vi "Origin.vi"(0 "PortNumber":u8=7) -> (1 "Received String1":string="NG\r\n", 2 "Received String2":string, 3 "OK Done":bool)   [LabVIEW 2013]
panel:
  out "Received String Z 1":string="OK\r\n"
  in  "PortNumber Z":u8=8
  out "Received String Z 2":string
  out "OK Done Z":bool
  # "Port Number 0=COM1"
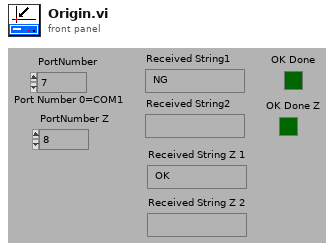
[diagram p1: front panel]
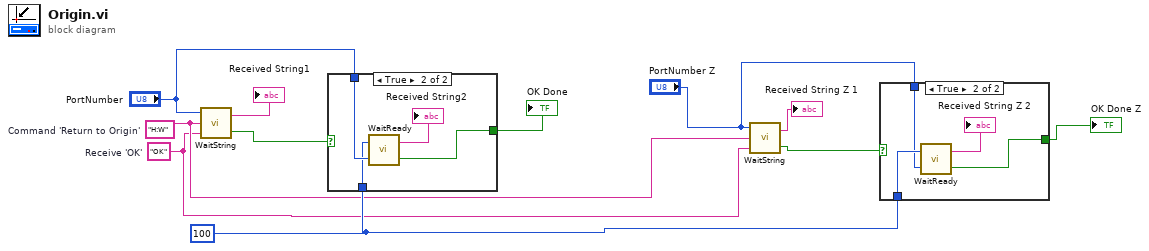
[diagram p0: block diagram]
diagram:
  w11 = 100
  w9 = "OK"  # Receive 'OK'
  w10 = "H:W"  # Command 'Return to Origin'
  n1 = call "WaitString.vi"("String to Receive"=w9, "String to Send"=w10, "PortNumber"="PortNumber") -> ("OK Done"=w5:bool, "String Received"=→"Received String1":string)
  n2 = case shown="True" w5 {
    selector: w5 -> [w12 _]
    tunnel: "PortNumber" -> [_ w16]
    tunnel: [w12 w14] -> w8
    tunnel: w11 -> [_ w13]
    frame False {
    }
    frame True {
      n3 = call "WaitReady.vi"("PortNumber"=w16, "Residence time in ms"=w13) -> ("OK Done"=w14:bool, "String Received"=→"Received String2":string)
    }
  }
  "OK Done" <- w8
  n4 = call "WaitString.vi"("String to Receive"=w9, "String to Send"=w10, "PortNumber"="PortNumber Z") -> ("OK Done"=w3:bool, "String Received"=→"Received String Z 1":string)
  n5 = case shown="True" w3 {
    selector: w3 -> [w17 _]
    tunnel: [w17 w20] -> w2
    tunnel: w11 -> [_ w19]
    tunnel: "PortNumber Z" -> [_ w18]
    frame False {
    }
    frame True {
      n6 = call "WaitReady.vi"("PortNumber"=w18, "Residence time in ms"=w19) -> ("OK Done"=w20:bool, "String Received"=→"Received String Z 2":string)
    }
  }
  "OK Done Z" <- w2
